vi "Export Image.vi"(0 "Display State In":T1, 5 "File Type":enum32{"BMP", "EPS", "EMF", "PICT"}(ring), 7 "Target":enum32{"File", "Clipboard"}(ring), 9 "Container State":T3, 11 "error in (no error)":errorcluster, 12 "Path":path, 13 "Hide Grid":bool, 14 "Always Overwrite":bool) -> (4 "Display State Out":T1, 15 "error out":errorcluster)   [LabVIEW 2017, in "2D Feather.xctl"]
uses:
  <vilib>/Math Plots/2D Math Plots/2D Feather/2D Feather XCtrl/2D Feather.xctl
  <vilib>/_xctls/Container State.ctl
  <vilib>/Math Plots/2D Math Plots/2D Feather/2D Feather XCtrl/State.ctl
  <vilib>/Math Plots/2D Math Plots/2D Feather/2D Feather/2D Feather.lvclass
  <vilib>/Math Plots/2D Math Plots/2D Plot/Action String/2DMathPlot Ctrl Act Queue.ctl
  <vilib>/Math Plots/2D Math Plots/2D Plot/Action String/2DMathPlot Ctrl Act Cluster.ctl
  <vilib>/Math Plots/2D Math Plots/2D Plot/Action String/2DMathPlot State Class.ctl
  <vilib>/_xctls/XControlSupport.lvlib
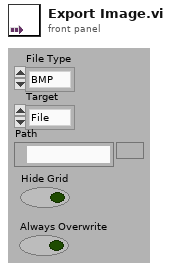
[diagram p1: front panel]
types:
  T1 = typedef "2D Feather.xctl/State.ctl" = cluster{"2D Feather.lvclass":refnum<class "2D Feather.lvclass">, "Control Ref Queue":T2, "Main Frame Color":u32, "Plot Legend Color":u32}
  T2 = typedef "2DMathPlot Ctrl Act Queue.ctl" = refnum<queue>
  T3 = typedef "XControlSupport.lvlib/Container State.ctl" = cluster{"Indicator?":bool, "Run Mode?":bool, " Refnum":refnum<vi>}
  T4 = typedef "2DMathPlot Ctrl Act Cluster.ctl" = cluster{"Plot Area Ref":refnum<vi>, "Z Axis Ref":refnum<vi>, "Legend Ref":refnum<vi>, "XControl Ref":refnum<vi>, "Facade Ref":refnum<vi>, "Display State Change Class":T5}
  T5 = typedef "2DMathPlot State Class.ctl" = enum16{"Update All (Undo)", "Update General", "Update Appearance", "Update Format", "Update Scale", "Update Marker", "Update Cursor", "None"}
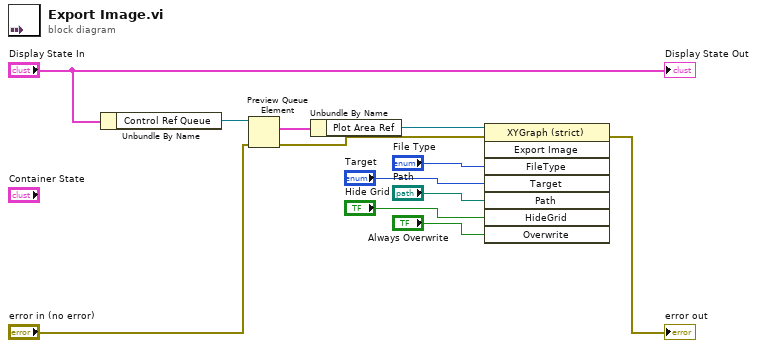
[diagram p0: block diagram]
diagram:
  n1 = Unbundle By Name("Display State In") -> ("Control Ref Queue"=w11:T2)
  n2 = Preview Queue Element(queue=w11, error in (no error)="error in (no error)") -> (element=w10:T4, error out=w3:errorcluster)  [unwired: 3 out]
  n3 = Unbundle By Name(w10) -> ("Plot Area Ref"=w9:refnum<vi>)
  n4 = invoke class="XYGraph (strict)" method="Export Image"(reference=w9, error in=w3, "FileType"="File Type", "Target"="Target", "Path"="Path", "HideGrid"="Hide Grid", "Overwrite"="Always Overwrite") -> (error out=→"error out":errorcluster)  [unwired: 1 in, 7 out]
  "Display State Out" <- "Display State In"
